vi "get desired keys.vi"(8 "error in":errorcluster, 11 "ExampleSequencer configuration in":refnum<class "ExampleSequencer configuration.lvclass">) -> (0 "error out":errorcluster, 2 "desired keys":string[](array[string]), 3 "ExampleSequencer configuration out":refnum<class "ExampleSequencer configuration.lvclass">)   [LabVIEW 2017, in "ExampleSequencer configuration.lvclass"]
uses:
  ExampleSequencer configuration.lvclass
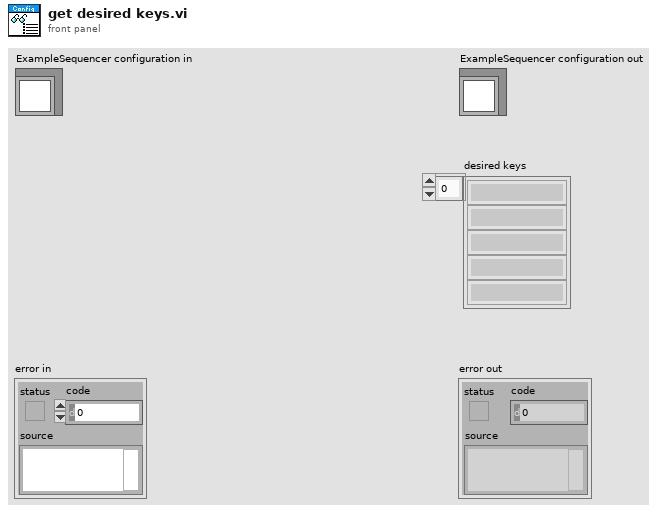
[diagram p1: front panel]
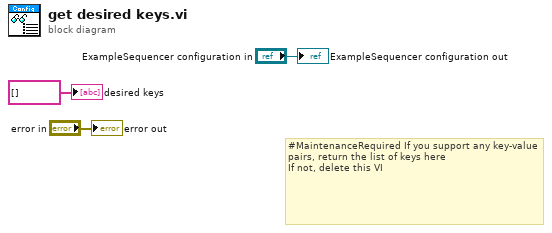
[diagram p0: block diagram]
diagram:
  # "#MaintenanceRequired If you support any key-value pairs, return the list of keys here\nIf not, delete this VI"
  "error out" <- "error in"
  "ExampleSequencer configuration out" <- "ExampleSequencer configuration in"
  "desired keys" <- string[] [] ("desired keys")
